vi "add cmag scan position(SubVI).vi"(10 "字符串":string) -> (0 "布尔 3":bool, 2 "连接的字符串":string)   [LabVIEW 2019, in "Add Seq.lvlib"]
uses:
  Add Seq.lvlib
panel:
  in  "轴向":enum16{"in plane", "out plane"}(ring)
  in  "Number of Step":i32=2
  in  "Step Delay(secs)":dbl
  in  "Increments":dbl=10.0
  in  "cancel":bool
  in  "ok":bool
  in  "Final Position":dbl min=-140000.0 max=140000.0
  in  "Initial Position":dbl min=-140000.0 max=140000.0
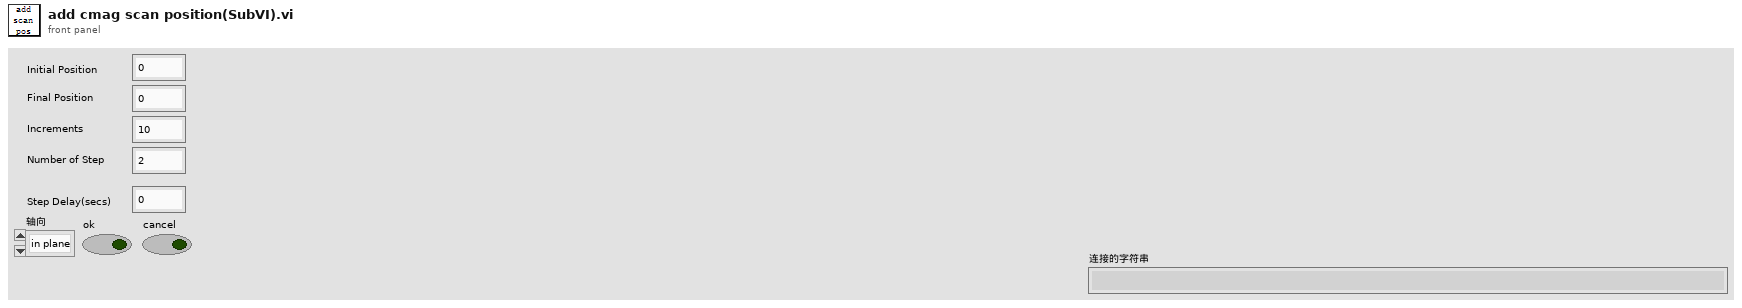
[diagram p1: front panel]
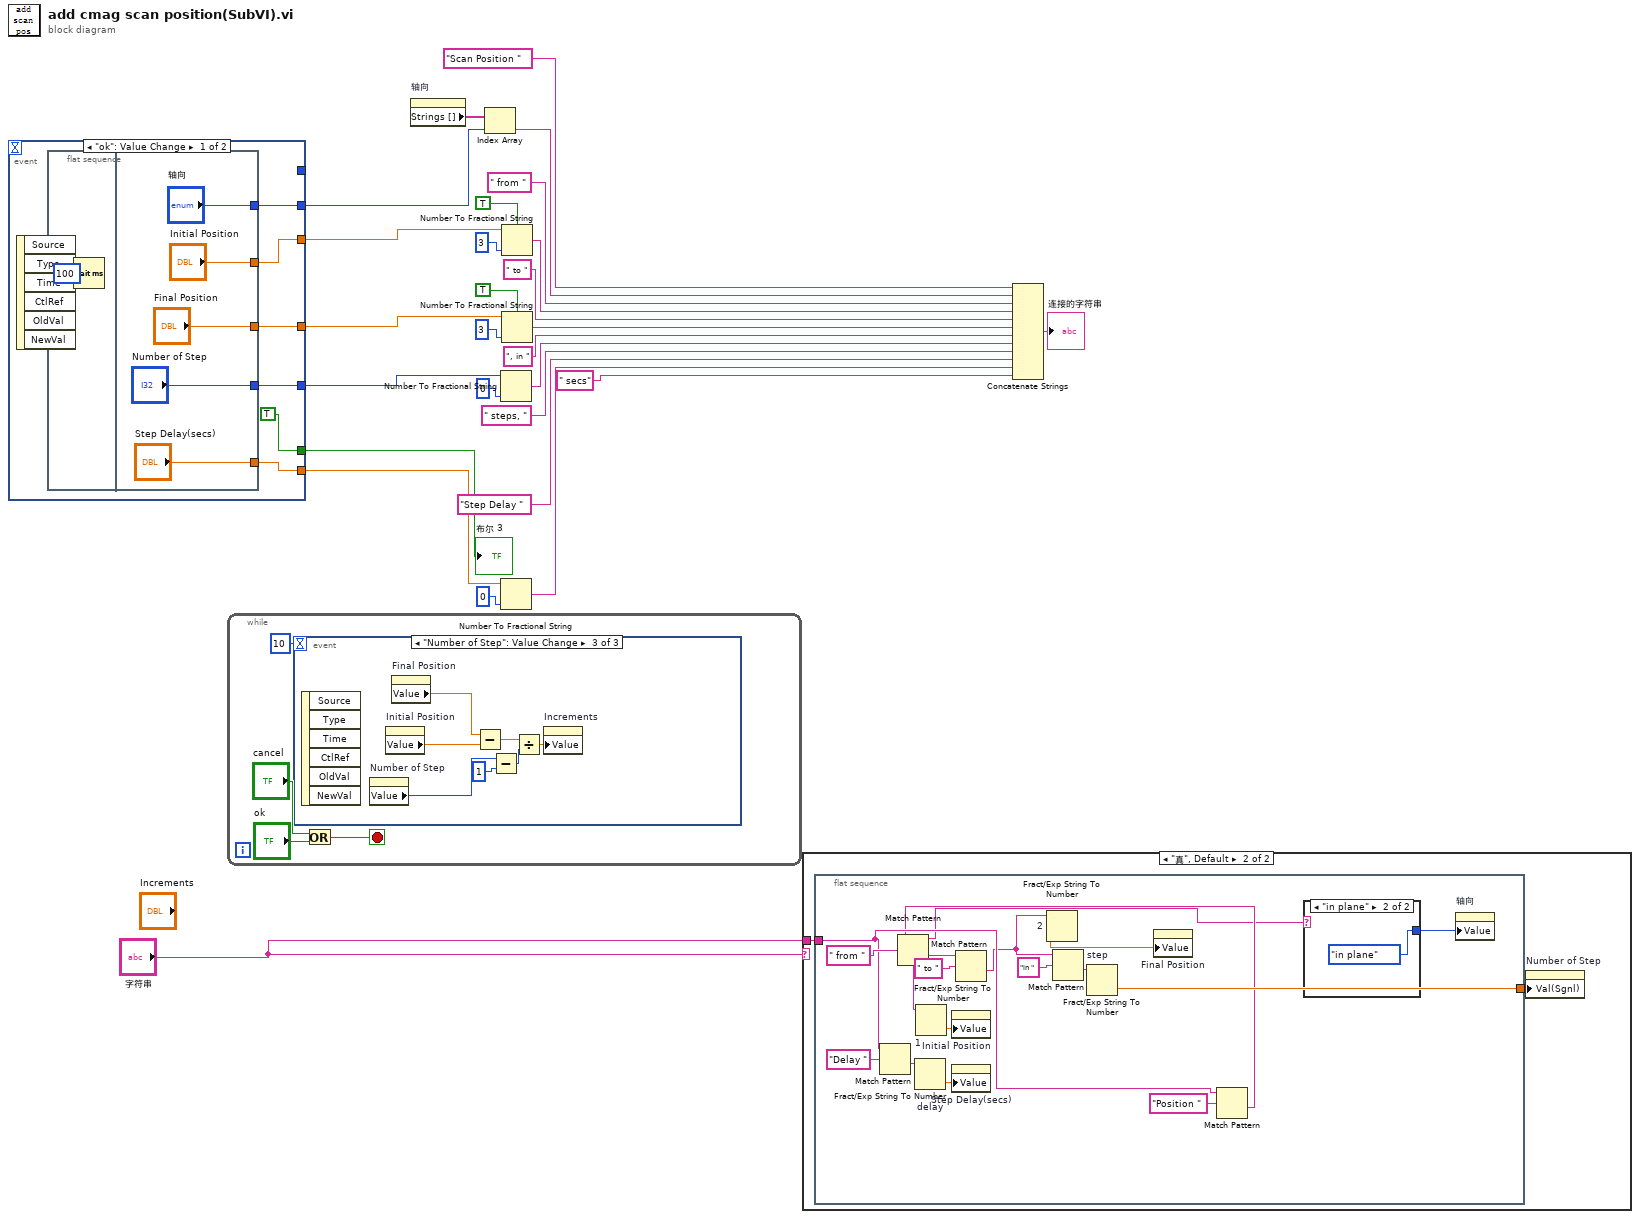
[diagram p0: block diagram]
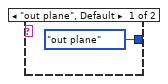
[diagram p3: hidden frame]
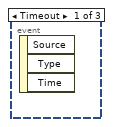
[diagram p4: hidden frame]
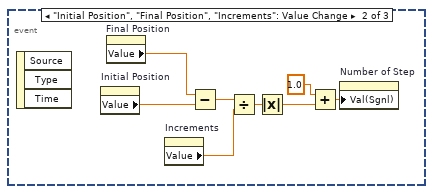
[diagram p5: hidden frame]
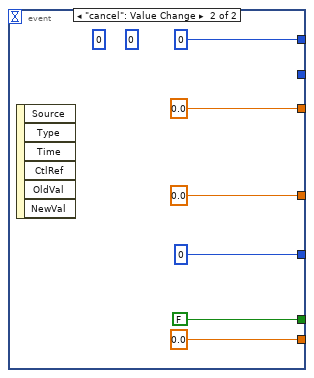
[diagram p6: hidden frame]
diagram:
  n1 = event shown="[0] \"ok\": Value Change" {
    selector: _ -> [_ _]
    dyn-events: _ -> [_ _]
    timeout: _ -> [_ _]
    tunnel: [w33 0.0 ("Field 2")] -> w17
    tunnel: [_ 0 ("Rate输入")] -> _
    tunnel: [w32 0.0 ("Field")] -> w25
    tunnel: [TRUE FALSE] -> w27
    tunnel: [w29 0 ("Number of Step")] -> w15
    tunnel: [w30 0.0 ("Step Delay(secs)")] -> w9
    tunnel: [w28 _] -> w1
    event "ok": Value Change {
      n2 = event-data() -> ()  [unwired: 1 in, 6 out]
      n3 = flat-sequence {
        tunnel: ["Final Position"] -> w33
        tunnel: ["Initial Position"] -> w32
        tunnel: ["Step Delay(secs)"] -> w30
        tunnel: ["Number of Step"] -> w29
        tunnel: ["轴向"] -> w28
        frame #0 {
          n4 = Wait (ms)(milliseconds to wait=u32 100) -> ()  [unwired: 1 out]
        }
        frame #1 {
        }
      }
    }
    event "cancel": Value Change {
      (unwired) 0 ("Approach")
      (unwired) 0 ("Approach输入")
      n5 = event-data() -> ()  [unwired: 1 in, 6 out]
    }
  }
  "布尔 3" <- w27
  n6 = while {
    stop <- w46 stop-if-true
    n7 = event shown="[2] \"Number of Step\": Value Change" {
      selector: _ -> [_ _ _]
      dyn-events: _ -> [_ _ _]
      timeout: 10 -> [_ _ _]
      event Timeout {
        n8 = event-data() -> ()  [unwired: 1 in, 3 out]
      }
      event "Initial Position", "Final Position", "Increments": Value Change {
        n9 = event-data() -> ()  [unwired: 1 in, 3 out]
        n10 = property on="Initial Position" class="DigNum (strict)"() -> ("Value"=w56:dbl)  [unwired: 2 in, 2 out]
        n11 = property on="Final Position" class="DigNum (strict)"() -> ("Value"=w57:dbl)  [unwired: 2 in, 2 out]
        n12 = property on="Increments" class="DigNum (strict)"() -> ("Value"=w54:dbl)  [unwired: 2 in, 2 out]
        n13 = Subtract(x=w57, y=w56) -> (x-y=w55:dbl)
        n14 = Divide(x=w55, y=w54) -> (x/y=w51:dbl)
        n15 = Absolute Value(x=w51) -> (abs(x)=w50:dbl)
        n16 = Add(x=1.0, y=w50) -> (x+y=w52:dbl)
        n17 = property on="Number of Step" class="DigNum (strict)"("Val(Sgnl)"=w52) -> ()  [unwired: 2 in, 2 out]
      }
      event "Number of Step": Value Change {
        n18 = event-data() -> ()  [unwired: 1 in, 6 out]
        n19 = property on="Number of Step" class="DigNum (strict)"() -> ("Value"=w61:i32)  [unwired: 2 in, 2 out]
        n20 = property on="Initial Position" class="DigNum (strict)"() -> ("Value"=w63:dbl)  [unwired: 2 in, 2 out]
        n21 = property on="Final Position" class="DigNum (strict)"() -> ("Value"=w64:dbl)  [unwired: 2 in, 2 out]
        n22 = Subtract(x=w64, y=w63) -> (x-y=w62:dbl)
        n23 = Subtract(x=w61, y=1) -> (x-y=w59:i32)
        n24 = Divide(x=w62, y=w59) -> (x/y=w58:dbl)
        n25 = property on="Increments" class="DigNum (strict)"("Value"=w58) -> ()  [unwired: 2 in, 2 out]
      }
    }
    n26 = Or(x="cancel", y="ok") -> (x .or. y?=w46:bool)
  }
  n27 = property on="轴向" class="Enum (strict)"() -> ("Strings []"=w4:string[])  [unwired: 2 in, 2 out]
  n28 = Index Array(array=w4, index=w1) -> (element=w3:string)
  n29 = Number To Fractional String(number=w15, precision (6)=i16 0 ("精度(6)")) -> (F-format string=w14:string)  [unwired: 2 in]
  n30 = Number To Fractional String(number=w9, precision (6)=i16 0 ("精度(6)")) -> (F-format string=w8:string)  [unwired: 2 in]
  n31 = Number To Fractional String(use system decimal point (T)=TRUE ("使用系统小数点(T)"), number=w25, precision (6)=i16 3 ("精度(6)")) -> (F-format string=w23:string)  [unwired: 1 in]
  n32 = Number To Fractional String(use system decimal point (T)=TRUE ("使用系统小数点(T)"), number=w17, precision (6)=i16 3 ("精度(6)")) -> (F-format string=w18:string)  [unwired: 1 in]
  n33 = case shown="\"真\", Default" "字符串" {
    tunnel: "字符串" -> [_ w66]
    frame "" {
    }
    frame "真", Default {
      n34 = flat-sequence {
        tunnel: w66 -> [w71]
        tunnel: [w73] -> w65
        frame #0 {
          n35 = Match Pattern(string=w71, regular expression="Delay " ("正则表达式")) -> (after substring=w81:string)  [unwired: 1 in, 3 out]
          n36 = Fract/Exp String To Number "delay"(string=w81) -> (number=w79:dbl)  [unwired: 3 in, 1 out]
          n37 = property on="Step Delay(secs)" class="DigNum (strict)"("Value"=w79) -> ()  [unwired: 2 in, 2 out]
          n38 = Match Pattern(string=w71, regular expression="Position " ("正则表达式")) -> (after substring=w70:string)  [unwired: 1 in, 3 out]
          n39 = Match Pattern(string=w70, regular expression=" from " ("正则表达式")) -> (before substring=w69:string, after substring=w78:string)  [unwired: 1 in, 2 out]
          n40 = Fract/Exp String To Number "1"(string=w78) -> (number=w80:dbl)  [unwired: 3 in, 1 out]
          n41 = property on="Initial Position" class="DigNum (strict)"("Value"=w80) -> ()  [unwired: 2 in, 2 out]
          n42 = Match Pattern(string=w78, regular expression=" to " ("正则表达式")) -> (after substring=w67:string)  [unwired: 1 in, 3 out]
          n43 = Fract/Exp String To Number "2"(string=w67) -> (number=w76:dbl)  [unwired: 3 in, 1 out]
          n44 = Match Pattern(string=w67, regular expression="in " ("正则表达式")) -> (after substring=w74:string)  [unwired: 1 in, 3 out]
          n45 = Fract/Exp String To Number "step"(string=w74) -> (number=w73:dbl)  [unwired: 3 in, 1 out]
          n46 = property on="Final Position" class="DigNum (strict)"("Value"=w76) -> ()  [unwired: 2 in, 2 out]
          n47 = case shown="\"in plane\"" w69 {
            tunnel: [enum16{"in plane", "out plane"}."out plane" ("轴向") enum16{"in plane", "out plane"}."in plane" ("轴向")] -> w68
            frame "out plane", Default {
            }
            frame "in plane" {
            }
          }
          n48 = property on="轴向" class="Enum (strict)"("Value"=w68) -> ()  [unwired: 2 in, 2 out]
        }
      }
      n49 = property on="Number of Step" class="DigNum (strict)"("Val(Sgnl)"=w65) -> ()  [unwired: 2 in, 2 out]
    }
  }
  n50 = Concatenate Strings("Scan Position " ("字符串"), w3, " from " ("字符串"), w23, " to " ("字符串"), w18, ", in " ("字符串"), w14, " steps, " ("字符串"), "Step Delay " ("字符串"), w8, " secs" ("字符串")) -> (→"连接的字符串":string)
